vi "process.vi"(8 "error in (no error)":errorcluster, 10 "Sync":refnum<notifier>, 11 "Session in":refnum<class "Session.lvclass">) -> (0 "error out":errorcluster, 3 "Session out":refnum<class "Session.lvclass">)   [LabVIEW 2013, in "MQTT Base.lvlib" / "Session.lvclass"]
uses:
  Session.lvclass
  Session.lvclass/Session.ctl
  <vilib>/LabVIEW Open Source Project/MQTT Control Packets/Control Packets/ControlPacket/ControlPacket.lvclass
  <vilib>/LabVIEW Open Source Project/MQTT Control Packets/Control Packets/MQTT_311/MQTTVersion.lvclass
  MQTT_Connection/Connection/Connection.lvclass
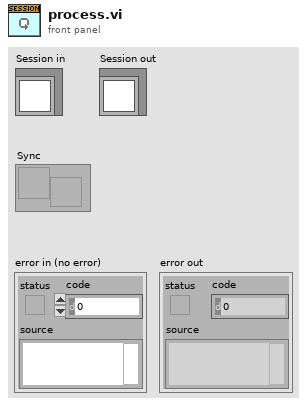
[diagram p1: front panel]
types:
  T1 = typedef "MQTT Base.lvlib/MQTT_Base.lvclass/Response -- cluster.ctl" = cluster{"Packet":refnum<class "ControlPacket.lvclass">, "Protocol Error":errorcluster, "disconnect session":bool, "[ACK]":refnum<notifier>[]}
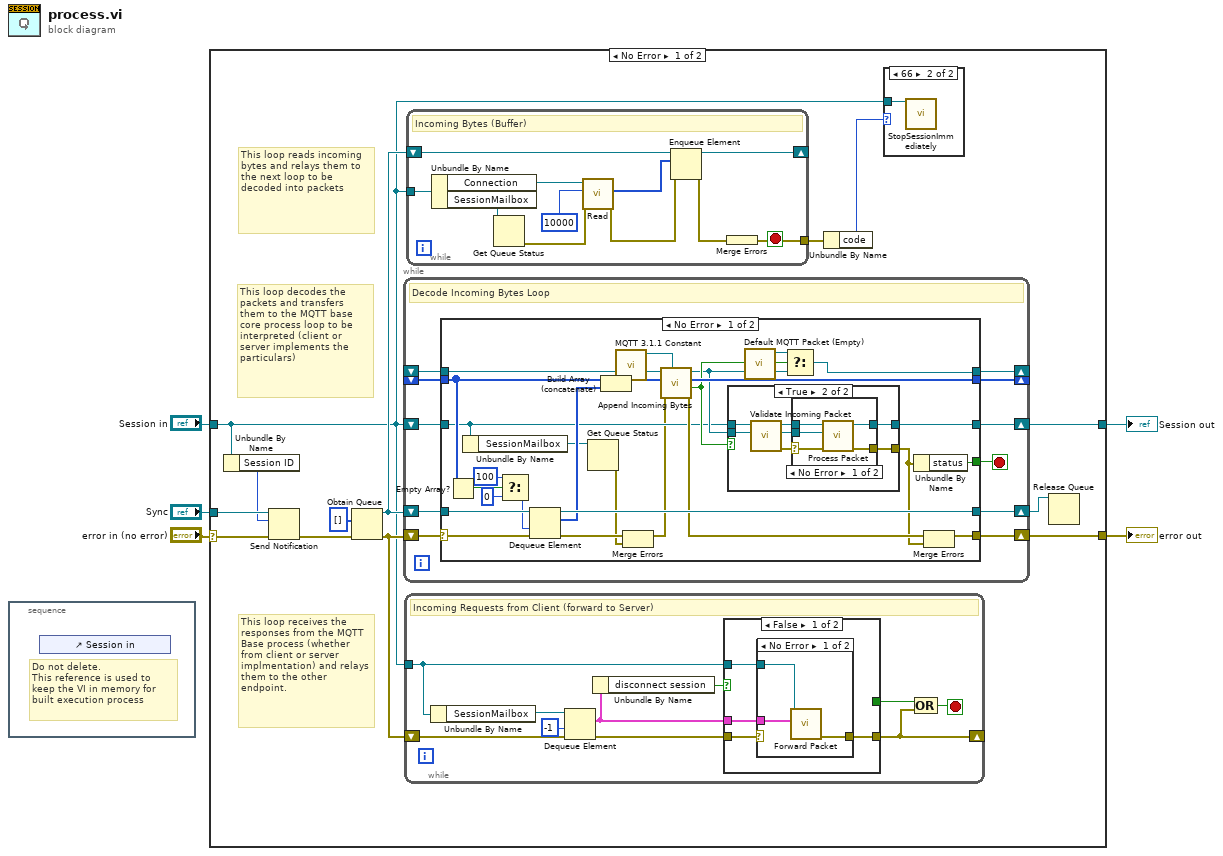
[diagram p0: block diagram]
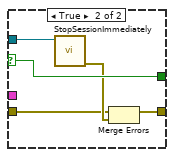
[diagram p3: hidden frame]
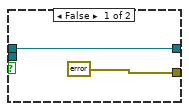
[diagram p5: hidden frame]
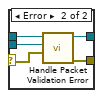
[diagram p6: hidden frame]
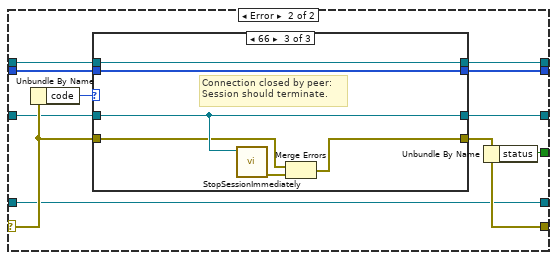
[diagram p7: hidden frame]
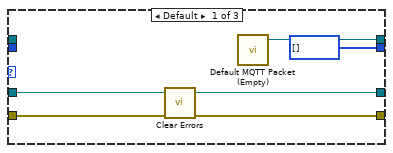
[diagram p8: hidden frame]
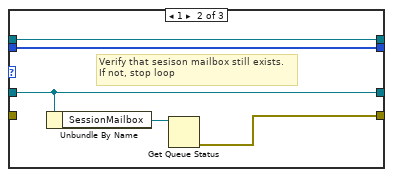
[diagram p9: hidden frame]
diagram:
  n1 = stacked-sequence {
    frame #0 {
      # "Do not delete.\nThis reference is used to keep the VI in memory for built execution process"
      n2 = control-ref of="Session in"() -> ()  [unwired: 1 out]
    }
  }
  n3 = case shown="No Error" "error in (no error)" {
    selector: "error in (no error)" -> [w17 w139]
    tunnel: [w8 w139] -> w1
    tunnel: [w11 w138] -> w3
    tunnel: "Session in" -> [w7 w138]
    tunnel: "Sync" -> [w18 _]
    frame No Error {
      # "This loop receives the responses from the MQTT Base process (whether from client or server implmentation) and relays them to the other endpoint."
      # "This loop decodes the packets and transfers them to the MQTT base core process loop to be interpreted (client or server implements the particulars)"
      # "This loop reads incoming bytes and relays them to the next loop to be decoded into packets"
      n4 = Unbundle By Name(w7) -> ("Session ID"=w6:i32)
      n5 = Send Notification(notification=w6, notifier=w18, error in (no error)=w17) -> (error out=w10:errorcluster)  [unwired: 1 out]
      n6 = Obtain Queue(element data type=u8[] [] ("Remaining Packets"), error in (no error)=w10) -> (queue out=w13:refnum<queue>, error out=w16:errorcluster)  [unwired: 3 in, 1 out]
      n7 = while {
        shift-right: [w62] -> _
        shift-left: _ -> [w61]
        shift-right: [w60] -> w8
        shift-left: w16 -> [w59]
        shift-right: [w63] -> _
        shift-left: _ -> [w64]
        shift-right: [w56] -> w9
        shift-left: w13 -> [w57]
        shift-right: [w54] -> w11
        shift-left: w7 -> [w55]
        stop <- w58 stop-if-true
        # "Decode Incoming Bytes Loop"
        n8 = case shown="No Error" w59 {
          selector: w59 -> [w84 w119]
          tunnel: w64 -> [w91 w117]
          tunnel: [w76 w121] -> w63
          tunnel: [w89 w120] -> w62
          tunnel: w61 -> [w81 w111]
          tunnel: [w82 w116] -> w60
          tunnel: [w70 w115] -> w58
          tunnel: w57 -> [w88 w114]
          tunnel: [w87 w114] -> w56
          tunnel: w55 -> [w69 w113]
          tunnel: [w72 w112] -> w54
          frame No Error {
            # "No Error"
            n9 = Empty Array?(array=w81) -> (empty?=w80:bool)
            n10 = Unbundle By Name(w69) -> ("SessionMailbox"=w68:refnum<queue>)
            n11 = Select(t=100 ("timeout in ms (-1)"), s=w80, f=0) -> (s? t:f=w78:i32)
            n12 = Dequeue Element(queue=w88, timeout in ms (-1)=w78, error in (no error)=w84) -> (queue out=w87:refnum<queue>, element=w86:u8[], error out=w67:errorcluster)  [unwired: 1 out]
            n13 = Get Queue Status(queue=w68) -> (error out=w66:errorcluster)  [unwired: 2 in, 7 out]
            n14 = Build Array (concatenate)(w81, w86) -> (w85:u8[])
            n15 = call <vilib>:"MQTT 3.1.1 Constant.vi"() -> ("MQTT 3.1.1"=w90:refnum<class "MQTTVersion.lvclass">)  [unwired: 11 in]
            n16 = Merge Errors(w67, w66) -> (w65:errorcluster)
            n17 = call <vilib>:"Append Incoming Bytes.vi"("MQTT Version (3.1.1)"=w90, "error in (no error)"=w65, "Incoming Packets"=w85, "Incomplete ControlPacket"=w91) -> ("error out"=w83:errorcluster, "Complete Packet"=w74:bool, "Remaining Packets"=w89:u8[], "ControlPacket"=w73:refnum<class "ControlPacket.lvclass">)  [unwired: 4 in]
            n18 = case shown="True" w74 {
              tunnel: [errorcluster {"status"=FALSE, "code"=0, "source"=""} ("error out") w94] -> w71
              tunnel: w73 -> [_ w100]
              tunnel: w69 -> [w92 w99]
              tunnel: [w92 w95] -> w72
              frame False {
                # "No Packet received"
              }
              frame True {
                # "Packet Received"
                n19 = call-dynamic "Validate Incoming Packet.vi"("ControlPacket"=w100, "Session in"=w99) -> ("error out"=w96:errorcluster, "ControlPacket out"=w97:refnum<class "ControlPacket.lvclass">, "Session out"=w98:refnum<class "Session.lvclass">)  [unwired: 7 in]
                n20 = case shown="No Error" w96 {
                  selector: w96 -> [w101 w108]
                  tunnel: [w102 w106] -> w95
                  tunnel: w98 -> [w105 w110]
                  tunnel: w97 -> [w104 w109]
                  tunnel: [w103 w107] -> w94
                  frame No Error {
                    n21 = call-dynamic "Process Packet.vi"("error in (no error)"=w101, "Incoming Packet"=w104, "Session in"=w105) -> ("error out"=w103:errorcluster, "Session out"=w102:refnum<class "Session.lvclass">)  [unwired: 7 in]
                  }
                  frame Error {
                    n22 = call "Handle Packet Validation Error.vi"("Packet Validation Error"=w108, "ControlPacket"=w109, "Session in"=w110) -> ("error out"=w107:errorcluster, "Session out"=w106:refnum<class "Session.lvclass">)  [unwired: 7 in]
                  }
                }
              }
            }
            n23 = call <vilib>:"Default MQTT Packet (Empty).vi"() -> ("No Packet"=w75:refnum<class "ControlPacket.lvclass">)  [unwired: 11 in]
            n24 = Select(t=w75, s=w74, f=w73) -> (s? t:f=w76:refnum<class "ControlPacket.lvclass">)
            n25 = Unbundle By Name(w71) -> ("status"=w70:bool)
            n26 = Merge Errors(w83, w71) -> (w82:errorcluster)
          }
          frame Error {
            # "Handle Error"
            n27 = Unbundle By Name(w119) -> ("code"=w118:i32)
            n28 = case shown="66" w118 {
              tunnel: [w123 w130 w137] -> w121
              tunnel: w119 -> [w126 _ w133]
              tunnel: [w125 w127 w132] -> w116
              tunnel: [u8[] [] ("Remaining Packets") w129 w136] -> w120
              tunnel: w117 -> [_ w130 w137]
              tunnel: w113 -> [w122 w128 w135]
              tunnel: [w122 w128 w135] -> w112
              tunnel: w111 -> [_ w129 w136]
              frame Default {
                # "Malformed Packet"
                n29 = call <vilib>:"Clear Errors.vi"("error in (no error)"=w126) -> ("error out"=w125:errorcluster)  [unwired: 6 in]
                n30 = call <vilib>:"Default MQTT Packet (Empty).vi"() -> ("No Packet"=w123:refnum<class "ControlPacket.lvclass">)  [unwired: 11 in]
              }
              frame 1 {
                # "Verify that sesison mailbox still exists.\nIf not, stop loop"
                n31 = Unbundle By Name(w128) -> ("SessionMailbox"=w131:refnum<queue>)
                n32 = Get Queue Status(queue=w131) -> (error out=w127:errorcluster)  [unwired: 2 in, 7 out]
              }
              frame 66 {
                # "Connection closed by peer:\nSession should terminate."
                n33 = call "StopSessionImmediately.vi"("Session in"=w135) -> ("error out"=w134:errorcluster)  [unwired: 9 in, 1 out]
                n34 = Merge Errors(w133, w134) -> (w132:errorcluster)
              }
            }
            n35 = Unbundle By Name(w116) -> ("status"=w115:bool)
          }
        }
      }
      n36 = while {
        tunnel: w7 -> [w24]
        shift-right: [w21] -> _
        shift-left: w16 -> [w25]
        stop <- w20 stop-if-true
        # "Incoming Requests from Client (forward to Server)"
        n37 = Unbundle By Name(w24) -> ("SessionMailbox"=w28:refnum<queue>)
        n38 = Dequeue Element(queue=w28, timeout in ms (-1)=-1, error in (no error)=w25) -> (element=w23:T1, error out=w26:errorcluster)  [unwired: 2 out]
        n39 = Unbundle By Name(w23) -> ("disconnect session"=w22:bool)
        n40 = case shown="False" w22 {
          selector: w22 -> [_ w41]
          tunnel: w26 -> [w32 w38]
          tunnel: [w31 w37] -> w21
          tunnel: w24 -> [w30 w40]
          tunnel: w23 -> [w29 _]
          tunnel: [_ w41] -> w19
          frame False {
            n41 = case shown="No Error" w32 {
              selector: w32 -> [_ w36]
              tunnel: w29 -> [w34 _]
              tunnel: [w33 w36] -> w31
              tunnel: w30 -> [w35 _]
              frame No Error {
                n42 = call-dynamic "Forward Packet.vi"("Response"=w34, "Session in"=w35) -> ("error out"=w33:errorcluster)  [unwired: 9 in]
              }
              frame Error {
              }
            }
          }
          frame True {
            n43 = call "StopSessionImmediately.vi"("Session in"=w40) -> ("error out"=w39:errorcluster)  [unwired: 9 in, 1 out]
            n44 = Merge Errors(w38, w39) -> (w37:errorcluster)
          }
        }
        n45 = Compound Arithmetic op=OR(w19, w21) -> (w20:bool)
      }
      n46 = while {
        tunnel: w7 -> [w53]
        shift-right: [w50] -> _
        shift-left: w13 -> [w51]
        tunnel: [w48] -> w14
        stop <- w48 stop-if-true
        # "Incoming Bytes (Buffer)"
        n47 = Unbundle By Name(w53) -> ("Connection"=w47:refnum<class "Connection.lvclass">, "SessionMailbox"=w52:refnum<queue>)
        n48 = Get Queue Status(queue=w52) -> (error out=w44:errorcluster)  [unwired: 2 in, 7 out]
        n49 = call "Read.vi"("error in (no error)"=w44, "bytes to read (100)"=10000, "TCPConnection in"=w47) -> ("error out"=w43:errorcluster, "Bytes"=w46:u8[])  [unwired: 4 in, 3 out]
        n50 = Enqueue Element(queue=w51, element=w46, error in (no error)=w43) -> (queue out=w50:refnum<queue>, error out=w49:errorcluster)  [unwired: 1 in, 1 out]
        n51 = Merge Errors(w49) -> (w48:errorcluster)
      }
      n52 = Unbundle By Name(w14) -> ("code"=w15:i32)
      n53 = case shown="66" w15 {
        tunnel: w7 -> [_ w42]
        frame Default {
        }
        frame 66 {
          n54 = call "StopSessionImmediately.vi"("Session in"=w42) -> ()  [unwired: 9 in, 2 out]
        }
      }
      n55 = Release Queue(queue=w9) -> ()  [unwired: 2 in, 3 out]
    }
    frame Error {
    }
  }
  "error out" <- w1
  "Session out" <- w3
